vi "AMC Read Next Message.vi"(8 "error in (no error)":errorcluster, 9 "Termination List ([Exit])":string[](array[string])=["Exit"], 10 "timeout (1ms)":i32=1, 11 "Message Queue in":T3) -> (0 "error out":errorcluster, 1 "Message Value":string, 2 "Message Name":string, 3 "Message Queue out":T3, 4 "Message Attributes":T1, 5 "Exit Process":bool, 6 "Message":T2)   [LabVIEW 2012, in "REx_Springboard.lvlib" / "TLB_Dependencies.lvlib"]
doc: "This VI returns the next message from the message queue passed in. If the returned message matches any of the message names listed in the Termination List the Exit Process indicator will return True. If no message is available on the queue within the Timeout limit, the VI returns with the Timed Out indicator set True."
uses:
  TLB_Dependencies.lvlib
  amc_Message Queue.ctl
  amc_Message.ctl
  <vilib>/FTP/util/Keyed Array.ctl
  <vilib>/FTP/NI_FTP.lvlib
panel:
  out "Timed Out":bool
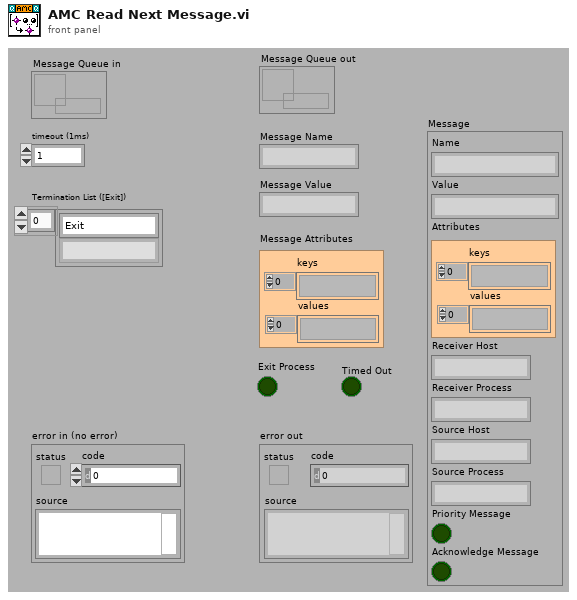
[diagram p1: front panel]
types:
  T1 = typedef "NI_FTP.lvlib/Keyed Array.ctl" = cluster{"keys":string[], "values":string[]}
  T2 = typedef "REx_Springboard.lvlib/TLB_Dependencies.lvlib/amc_Message.ctl" = cluster{"Name":string, "Value":string, "Attributes":T1, "Receiver Host":string, "Receiver Process":string, "Source Host":string, "Source Process":string, "Priority Message":bool, "Acknowledge Message":bool}
  T3 = typedef "REx_Springboard.lvlib/TLB_Dependencies.lvlib/amc_Message Queue.ctl" = refnum<queue>
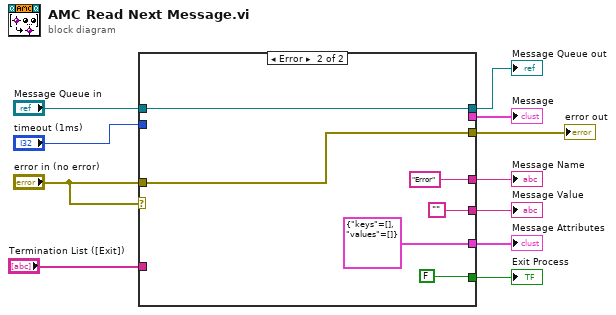
[diagram p0: block diagram]
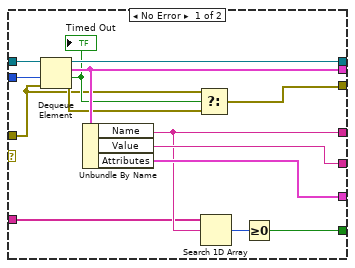
[diagram p2: hidden frame]
diagram:
  n1 = case shown="Error" "error in (no error)" {
    tunnel: "Message Queue in" -> [w25 w31]
    tunnel: [w24 w31] -> w7
    tunnel: [w19 "Error"] -> w9
    tunnel: "error in (no error)" -> [w12 w29]
    tunnel: "timeout (1ms)" -> [w23 _]
    tunnel: [w13 w29] -> w8
    tunnel: [w21 ""] -> w6
    tunnel: [w22 _] -> w4
    tunnel: [w20 T1 {"keys"=[], "values"=[]} ("Attributes")] -> w3
    tunnel: "Termination List ([Exit])" -> [w18 _]
    tunnel: [w16 FALSE] -> w1
    frame No Error {
      n2 = Dequeue Element(queue=w25, timeout in ms (-1)=w23, error in (no error)=w12) -> (queue out=w24:T3, element=w22:T2, timed out?=w15:bool, error out=w14:errorcluster)
      "Timed Out" <- w15
      n3 = Unbundle By Name(w22) -> ("Name"=w19:string, "Value"=w21:string, "Attributes"=w20:T1)
      n4 = Select(t=w12, s=w15, f=w14) -> (s? t:f=w13:errorcluster)
      n5 = Search 1D Array(1D array=w18, element=w19) -> (index of element=w17:i32)  [unwired: 1 out]
      n6 = Greater Or Equal To 0?(x=w17) -> (x >= 0?=w16:bool)
    }
    frame Error {
    }
  }
  "Message Queue out" <- w7
  "Message Name" <- w9
  "error out" <- w8
  "Message Value" <- w6
  "Message" <- w4
  "Message Attributes" <- w3
  "Exit Process" <- w1
